vi "remove_extra_space_character.vi"(8 "error in (no error)":errorcluster, 11 "Instrument Command In":string) -> (0 "error out":errorcluster, 3 "Instrument Command Out":string)   [LabVIEW 2018]
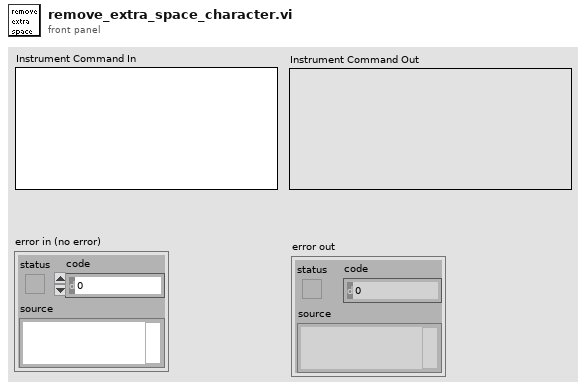
[diagram p1: front panel]
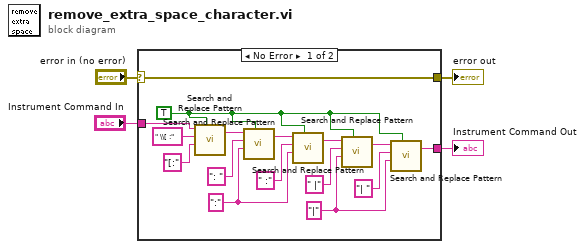
[diagram p0: block diagram]
diagram:
  n1 = case shown="No Error" "error in (no error)" {
    selector: "error in (no error)" -> [w11 w22]
    tunnel: "Instrument Command In" -> [w8 w21]
    tunnel: [w5 w21] -> w3
    tunnel: [w11 w22] -> w1
    frame No Error {
      w13 = "|"
      w6 = TRUE ("replace all? (F)")
      w20 = ":" ("replace string (\"\")")
      n2 = call <vilib>:"Search and Replace Pattern.vi"("string"=w8, "regular expression (\"\")"=" \\[ :" ("regular expression (\"\")"), "replace string (\"\")"="[:" ("replace string (\"\")"), "replace all? (F)"=w6) -> ("result string"=w7:string)  [unwired: 2 out]
      n3 = call <vilib>:"Search and Replace Pattern.vi"("string"=w7, "regular expression (\"\")"=": " ("regular expression (\"\")"), "replace string (\"\")"=w20, "replace all? (F)"=w6) -> ("result string"=w17:string)  [unwired: 2 out]
      n4 = call <vilib>:"Search and Replace Pattern.vi"("string"=w17, "regular expression (\"\")"=" :" ("regular expression (\"\")"), "replace string (\"\")"=w20, "replace all? (F)"=w6) -> ("result string"=w16:string)  [unwired: 2 out]
      n5 = call <vilib>:"Search and Replace Pattern.vi"("string"=w16, "regular expression (\"\")"=" |" ("regular expression (\"\")"), "replace string (\"\")"=w13, "replace all? (F)"=w6) -> ("result string"=w12:string)  [unwired: 2 out]
      n6 = call <vilib>:"Search and Replace Pattern.vi"("string"=w12, "regular expression (\"\")"="| " ("regular expression (\"\")"), "replace string (\"\")"=w13, "replace all? (F)"=w6) -> ("result string"=w5:string)  [unwired: 2 out]
    }
    frame Error {
    }
  }
  "Instrument Command Out" <- w3
  "error out" <- w1
